vi "EXA_Set_Trace_Type.vi"(8 "error in":errorcluster, 9 "Combo Box":string(combo), 10 "Trace\nNumber":i32, 11 "VISA resource name":refnum<visa-resource-name>) -> (0 "error out":errorcluster, 3 "VISA resource name":refnum<visa-resource-name>)   [LabVIEW 2016]
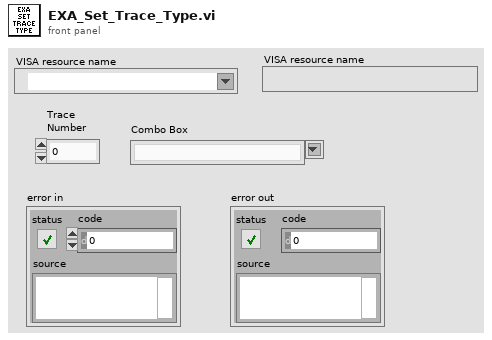
[diagram p1: front panel]
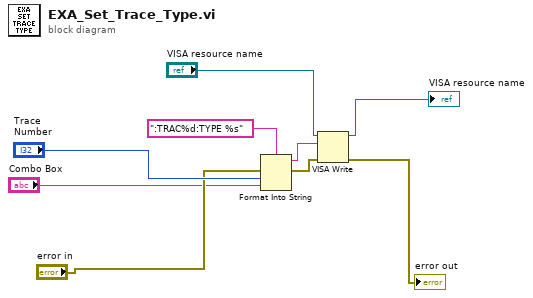
[diagram p0: block diagram]
diagram:
  n1 = Format Into String(format string=":TRAC%d:TYPE %s", error in="error in", "Trace\nNumber", "Combo Box") -> (resulting string=w4:string, error out=w7:errorcluster)  [unwired: 1 in]
  n2 = VISA Write(VISA resource name="VISA resource name", write buffer=w4, error in (no error)=w7) -> (VISA resource name out=→"VISA resource name":refnum<visa-resource-name>, error out=→"error out":errorcluster)  [unwired: 1 out]
